vi "Write States.vi"(8 "error in (no error)":errorcluster, 10 "States":enum16{"Exit", "AttackPs", "DefensePs"}(ring), 11 "DefaultPsTactic in":refnum<class "DefaultPsTactic.lvclass">) -> (0 "error out":errorcluster, 3 "DefaultPsTactic out":refnum<class "DefaultPsTactic.lvclass">)   [LabVIEW 2020, in "DefaultPsTactic.lvclass"]
uses:
  DefaultPsTactic.lvclass
  DefaultPsTactic.lvclass/DefaultPsTactic.ctl
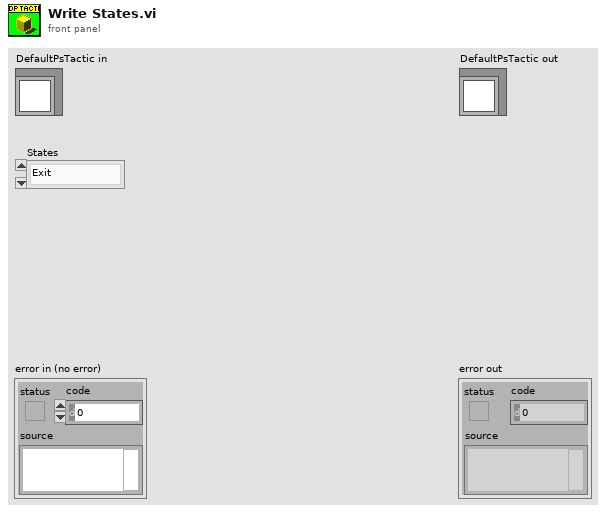
[diagram p1: front panel]
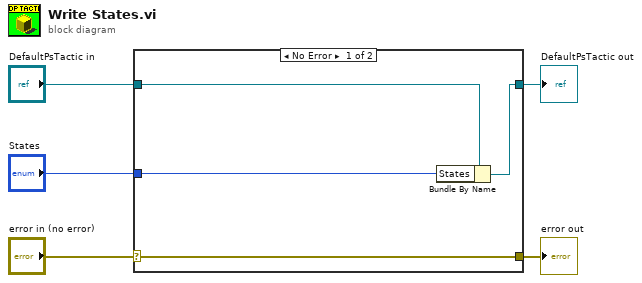
[diagram p0: block diagram]
diagram:
  n1 = case shown="No Error" "error in (no error)" {
    selector: "error in (no error)" -> [w9 w10]
    tunnel: [w9 w10] -> w4
    tunnel: [w7 w11] -> w2
    tunnel: "DefaultPsTactic in" -> [w8 w11]
    tunnel: "States" -> [w6 _]
    frame No Error {
      n2 = Bundle By Name(cluster=w8, "States"=w6) -> (w7:refnum<class "DefaultPsTactic.lvclass">)
    }
    frame Error {
    }
  }
  "error out" <- w4
  "DefaultPsTactic out" <- w2
